vi "Step Mode - Configure DC Voltage.vi"(8 "error in (no error)":errorcluster, 10 "DC Voltage":dbl, 11 "VISA resource name":refnum<visa-resource-name>) -> (0 "error out":errorcluster, 3 "VISA resource name out":refnum<visa-resource-name>)   [LabVIEW 2014, in "Associated Power Technologies 8500 Series.lvlib"]
doc: "Configure the basic DC voltage.\n\n<B>Note:</B>\nRange is AUTO: 0 ~ 420VDC\nRange is HIGH: 0 ~ 420VDC\nRange is LOW: 0 ~ 210VDC\n\nDefault value: 0 VDC"
uses:
  <instrlib>/Associated Power Technologies 8500 Series/Associated Power Technologies 8500 Series.lvlib
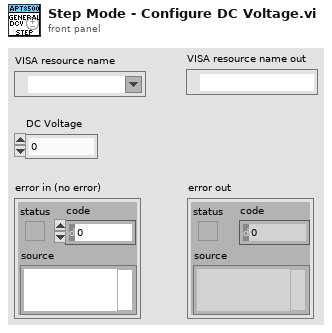
[diagram p1: front panel]
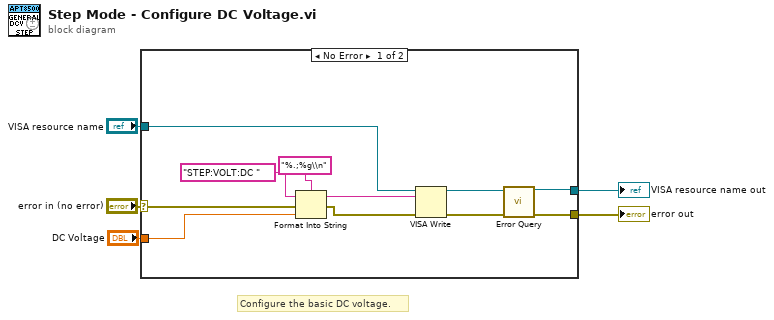
[diagram p0: block diagram]
diagram:
  # "Configure the basic DC voltage."
  n1 = case shown="No Error" "error in (no error)" {
    selector: "error in (no error)" -> [w15 w17]
    tunnel: "DC Voltage" -> [w16 _]
    tunnel: "VISA resource name" -> [w11 w18]
    tunnel: [w8 w18] -> w2
    tunnel: [w6 w17] -> w1
    frame No Error {
      n2 = Format Into String(format string="%.;%g\\n", initial string="STEP:VOLT:DC " ("command"), error in=w15, w16) -> (resulting string=w10:string, error out=w14:errorcluster)
      n3 = VISA Write(VISA resource name=w11, write buffer=w10, error in (no error)=w14) -> (VISA resource name out=w9:refnum<visa-resource-name>, error out=w7:errorcluster)  [unwired: 1 out]
      n4 = call <instrlib>:"Error Query.vi"("VISA resource name"=w9, "error in (no error)"=w7) -> ("VISA resource name out"=w8:refnum<visa-resource-name>, "error out"=w6:errorcluster)  [unwired: 10 in, 2 out]
    }
    frame Error {
    }
  }
  "VISA resource name out" <- w2
  "error out" <- w1
